vi "Destroy.vi"(8 "error in (no error)":errorcluster, 11 "Dummy Motor in":refnum<class "Dummy Motor.lvclass">) -> (0 "error out":errorcluster)   [LabVIEW 2015, in "Dummy Motor.lvclass"]
uses:
  Dummy Motor.lvclass
  Dummy Motor.lvclass/Dummy Motor.ctl
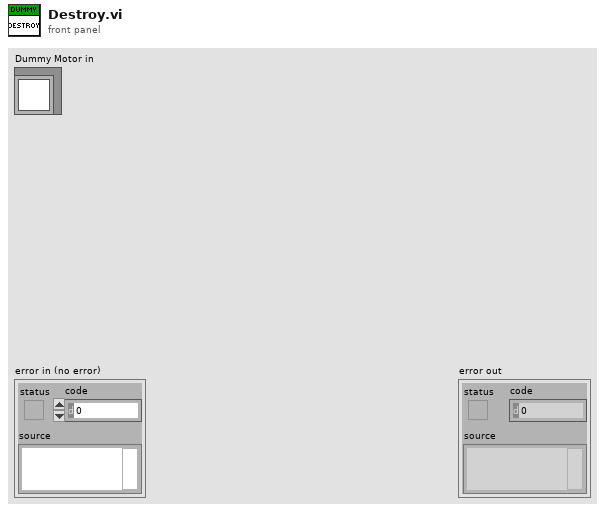
[diagram p1: front panel]
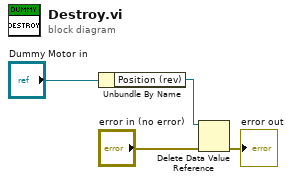
[diagram p0: block diagram]
diagram:
  n1 = Unbundle By Name("Dummy Motor in") -> ("Position (rev)"=w3:refnum<data-value>)
  n2 = Delete Data Value Reference(data value reference=w3, error in="error in (no error)") -> (error out=→"error out":errorcluster)  [unwired: 1 out]
